vi "Periodic Tasks.vi"(8 "error in":errorcluster) -> ()   [LabVIEW 2019]
doc: "This VI runs in parallel to other tasks. It can contain as many user-defined periodic loops as you need. These can carry out PID or other sorts of timed response."
uses:
  <vilib>/Rock Robotics/WPI/Utilities/WPI_GetSetVariantRefNum.vi
  Robot Global Data.vi
  <vilib>/addons/control/pid/pid.llb/PID (DBL).vi
  <vilib>/Rock Robotics/Network Tables/NT Write Numeric Array.vi
  <vilib>/Rock Robotics/Network Tables/NT Write Number.vi
  <vilib>/Rock Robotics/Network Tables/NT Write Boolean.vi
  Secret_Control_Library_Protected/Secret_Control_Library_Protected.lvlib
  <vilib>/addons/control/pid/NI_PID_pid.lvlib
  <vilib>/Rock Robotics/WPI/ThirdParty/JAS_Junk/TrajLib/Trajectory_Library.lvlib
panel:
  in  "Speed PID":T1={"proportional gain (Kc)"=0.6, "integral time (Ti, min)"=0.015, "derivative time (Td, min)"=0.0} {"derivative time (Td, min)" format="%.3f"; "integral time (Ti, min)" format="%.3f"; "proportional gain (Kc)" format="%.3f"}
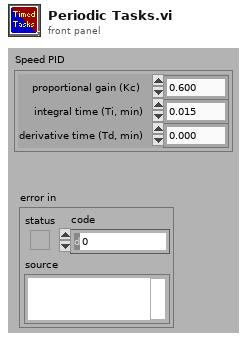
[diagram p1: front panel]
types:
  T1 = cluster{"proportional gain (Kc)":dbl, "integral time (Ti, min)":dbl, "derivative time (Td, min)":dbl}
  T2 = typedef "WPI_EncoderDevRef.ctl" = cluster{"DevStatus":errorcluster, "EncoderIndex":T3, "CounterIndex":T4, "DistancePerCount":dbl, "Decoding Type":T5}
  T3 = typedef "FPGA_EncoderIdx.ctl" = enum8{"Enc 0", "Enc 1", "Enc 2", "Enc 3", "Enc 4", "Enc 5", "Enc 6", "Enc 7", "Invalid"}
  T4 = typedef "FPGA_CounterCtrSystemIndex.ctl" = enum8{"Ctr 0", "Ctr 1", "Ctr 2", "Ctr 3", "Ctr 4", "Ctr 5", "Ctr 6", "Ctr 7", "Invalid"}
  T5 = typedef "WPI_EncoderType.ctl" = enum16{"1x", "2x", "4x"}
  T6 = typedef "WPI_GyroDevRef.ctl" = cluster{"DevStatus":errorcluster, "Analog Channel":T7, "Gain (VoltsPerDegree/Second)":dbl, "Gyro Type":enum16{"Analog", "XRS450"}, "Handle":i32, "SPI Bus":T8, "Device Found":bool, "Sample Rate":dbl, "Calibrate On Open":bool, "Offset":dbl}
  T7 = typedef "FPGA_AIChannel.ctl" = enum8{"AI 0", "AI 1", "AI 2", "AI 3", "AI MXP 0", "AI MXP 1", "AI MXP 2", "AI MXP 3", "Invalid"}
  T8 = typedef "spi_bus.ctl" = enum16{"SPI On-Board, CS0", "SPI On-Board, CS1", "SPI On-Board, CS2", "SPI On-Board, CS3", "SPI MXP", "Invalid"}
  T9 = typedef "WPI_RobotDriveDevRef.ctl" = cluster{"DevStatus":errorcluster, "Motors[]":T10[], "Square Inputs":bool, "Max Output":dbl}
  T10 = typedef "WPI_MotorControlDeviceRef.ctl" = cluster{"DeviceStatus":errorcluster, "Type":T11, "PWM":cluster{"PWM Channel":T12, "DeadBand":T13}, "CAN":cluster{"Device Number":u8, "SetOutput VI Ref":variant, "GetOutput VI Ref":variant, "Enable VI Ref":variant, "Disable VI Ref":variant, "Data":variant}, "Invert":bool, "DIO PWM":cluster{"PWM \"Enable\" Channel":T12, "DIOChannel":T14, "PWM Rate":dbl}}
  T11 = typedef "WPI_MotorControlType.ctl" = enum16{"PWM", "CAN", "DIO PWM"}
  T12 = typedef "FPGA_DIOPWMChannel.ctl" = enum8{"PWM 0", "PWM 1", "PWM 2", "PWM 3", "PWM 4", "PWM 5", "PWM 6", "PWM 7", "PWM 8", "PWM 9", "PWM MXP 0", "PWM MXP 1", "PWM MXP 2", "PWM MXP 3", "PWM MXP 4", "PWM MXP 5", "PWM MXP 6", "PWM MXP 7", "PWM MXP 8", "PWM MXP 9", "Invalid"}
  T13 = typedef "WPI_PWMDeadband.ctl" = cluster{"Name":string, "maxPositivePwm":i32, "minPositivePwm":i32, "centerPwm":i32, "maxNegativePwm":i32, "minNegativePwm":i32, "angularRange":u16}
  T14 = typedef "FPGA_DIOChannel.ctl" = enum8{"DIO 0", "DIO 1", "DIO 2", "DIO 3", "DIO 4", "DIO 5", "DIO 6", "DIO 7", "DIO 8", "DIO 9", "DIO MXP 0", "DIO MXP 1", "DIO MXP 2", "DIO MXP 3", "DIO MXP 4", "DIO MXP 5", "DIO MXP 6", "DIO MXP 7", "DIO MXP 8", "DIO MXP 9", "DIO MXP 10", "DIO MXP 11", "DIO MXP 12", "DIO MXP 13", "DIO MXP 14", "DIO MXP 15", "SPI Port CS1", "SPI Port CS2", "SPI Port CS3", "SPI Port MISO", "SPI Port MOSI", "Invalid"}
  T15 = typedef "Trajectory_Library.lvlib/SIMPLE_MOTOR_FF.ctl" = cluster{"Ks":dbl, "Kv":dbl, "Ka":dbl}
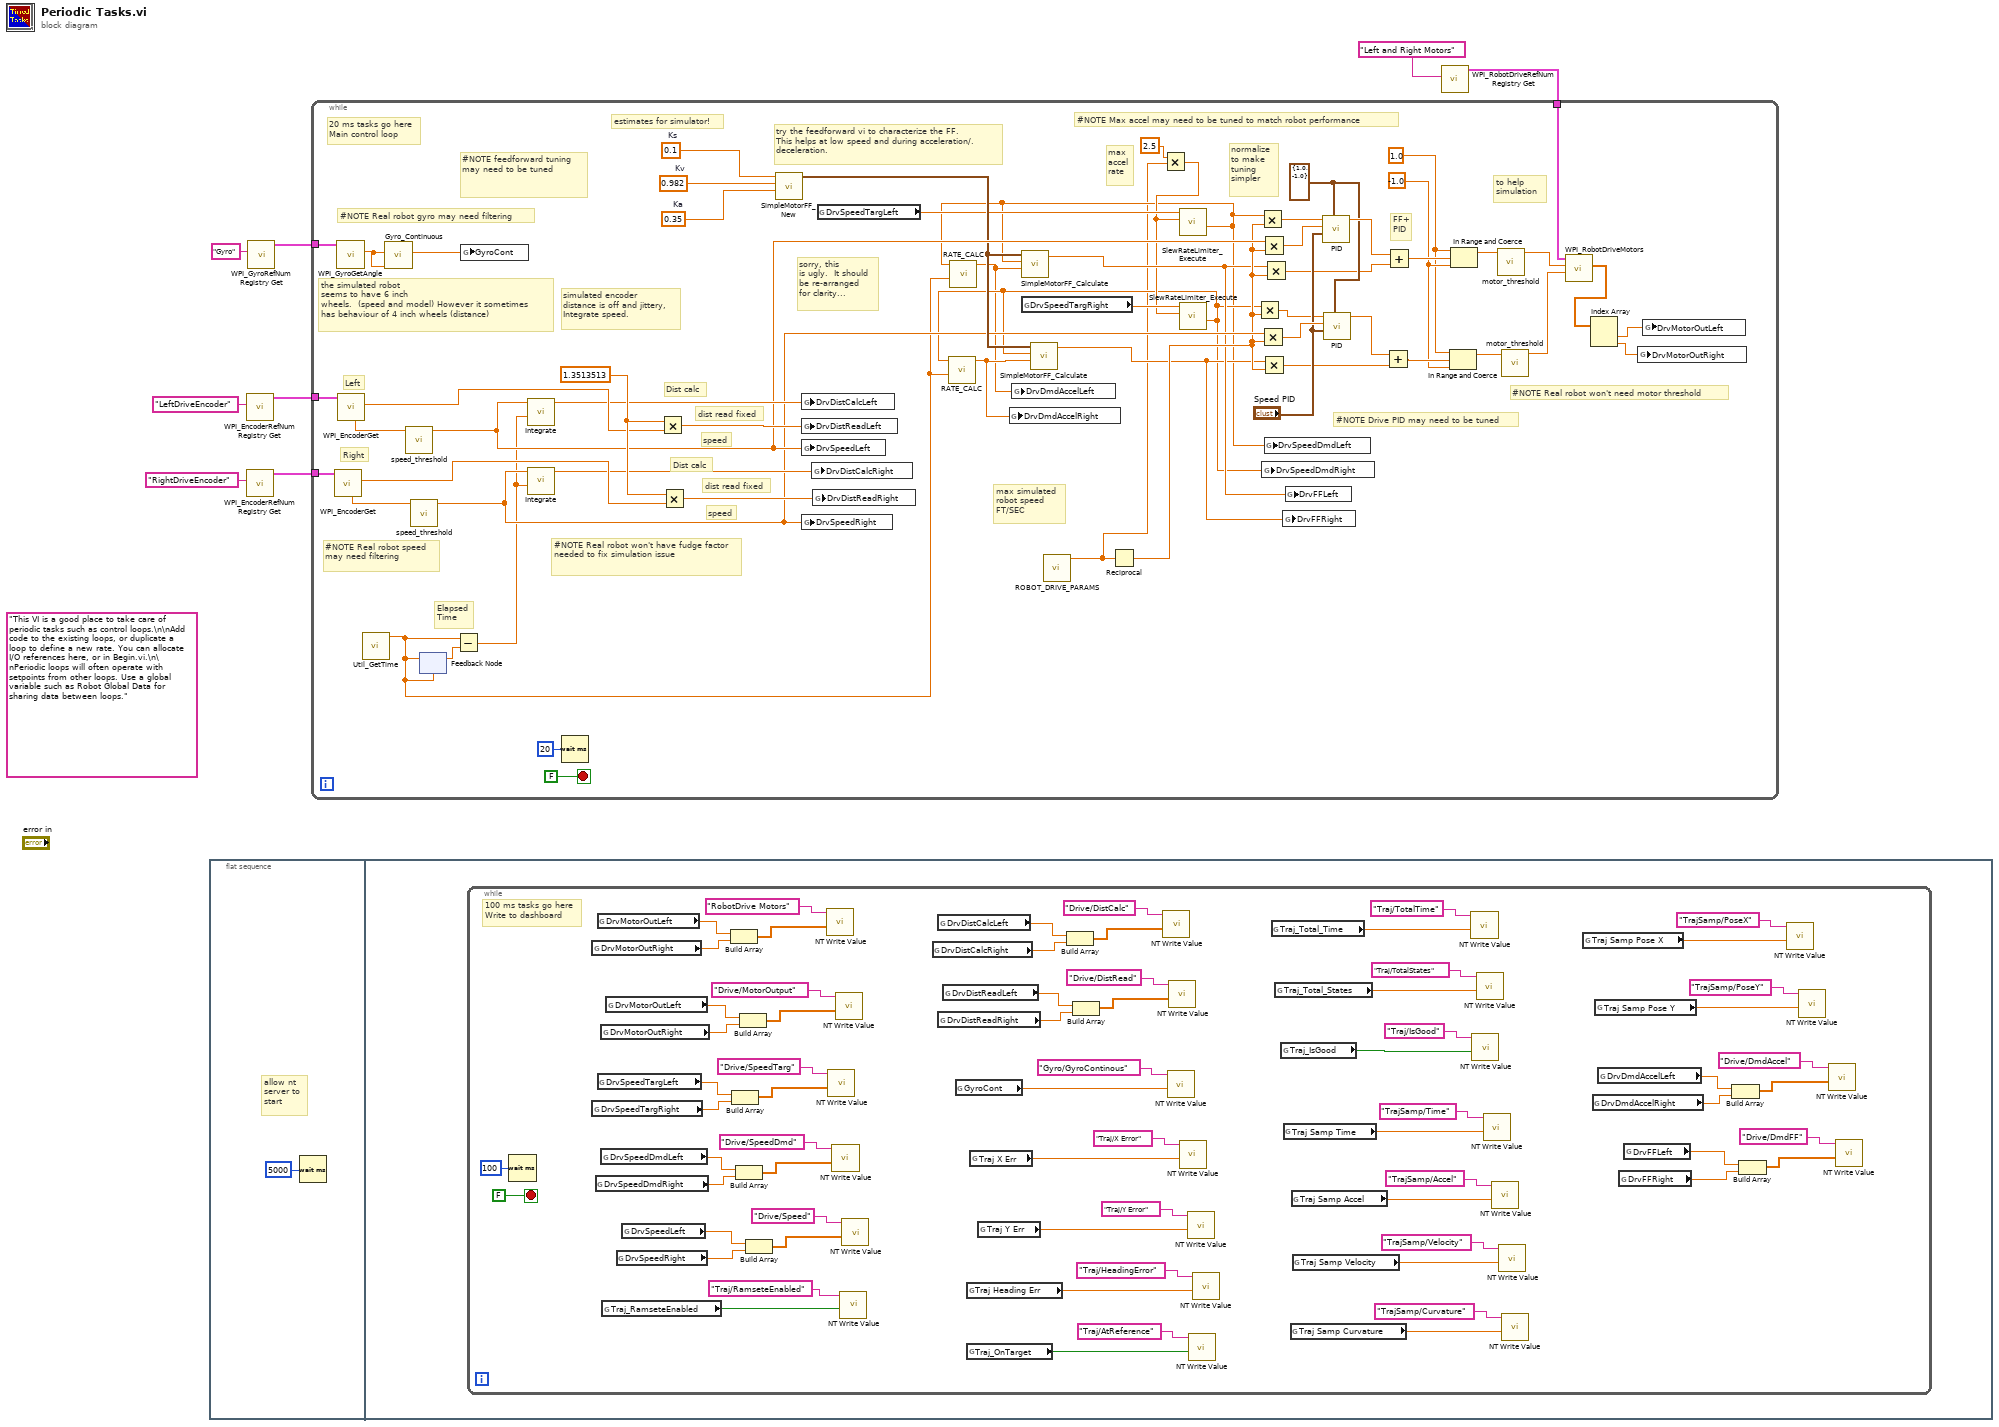
[diagram p0: block diagram]
diagram:
  (unwired) "This VI is a good place to take care of periodic tasks such as control loops.\n\nAdd code to the existing loops, or duplicate a loop to define a new rate. You can allocate I/O references here, or in Begin.vi.\n\nPeriodic loops will often operate with setpoints from other loops. Use a global variable such as Robot Global Data for sharing data between loops."
  n1 = flat-sequence {
    frame #0 {
      # "allow nt\nserver to \nstart"
      n2 = Wait (ms)(milliseconds to wait=u32 5000) -> ()  [unwired: 1 out]
    }
    frame #1 {
      n3 = while {
        stop <- FALSE stop-if-true
        # "100 ms tasks go here\nWrite to dashboard"
        n4 = Wait (ms)(milliseconds to wait=u32 100) -> ()  [unwired: 1 out]
        n5 = global read "Robot Global Data.vi" "DrvMotorOutRight"() -> (w74:dbl)
        n6 = global read "Robot Global Data.vi" "DrvSpeedTargRight"() -> (w66:dbl)
        n7 = global read "Robot Global Data.vi" "DrvSpeedDmdRight"() -> (w62:dbl)
        n8 = global read "Robot Global Data.vi" "DrvMotorOutLeft"() -> (w75:dbl)
        n9 = global read "Robot Global Data.vi" "DrvSpeedTargLeft"() -> (w67:dbl)
        n10 = global read "Robot Global Data.vi" "DrvMotorOutRight"() -> (w70:dbl)
        n11 = global read "Robot Global Data.vi" "DrvSpeedDmdLeft"() -> (w63:dbl)
        n12 = global read "Robot Global Data.vi" "Traj_RamseteEnabled"() -> (w11:bool)
        n13 = global read "Robot Global Data.vi" "DrvMotorOutLeft"() -> (w71:dbl)
        n14 = global read "Robot Global Data.vi" "DrvSpeedRight"() -> (w58:dbl)
        n15 = global read "Robot Global Data.vi" "DrvSpeedLeft"() -> (w59:dbl)
        n16 = Build Array(w75, w74) -> (w73:dbl[])
        n17 = Build Array(w67, w66) -> (w65:dbl[])
        n18 = Build Array(w63, w62) -> (w61:dbl[])
        n19 = Build Array(w71, w70) -> (w69:dbl[])
        n20 = Build Array(w59, w58) -> (w57:dbl[])
        n21 = call-poly <vilib>:"NT Write Value.vi"("Numeric Array"=w73, "Name"="RobotDrive Motors") -> ()  [unwired: 9 in, 1 out]
        n22 = call-poly <vilib>:"NT Write Value.vi"("Numeric Array"=w65, "Name"="Drive/SpeedTarg") -> ()  [unwired: 9 in, 1 out]
        n23 = call-poly <vilib>:"NT Write Value.vi"("Numeric Array"=w61, "Name"="Drive/SpeedDmd") -> ()  [unwired: 9 in, 1 out]
        n24 = call-poly <vilib>:"NT Write Value.vi"("Numeric Array"=w69, "Name"="Drive/MotorOutput") -> ()  [unwired: 9 in, 1 out]
        n25 = call-poly <vilib>:"NT Write Value.vi"("Boolean"=w11, "Name"="Traj/RamseteEnabled") -> ()  [unwired: 9 in, 1 out]
        n26 = call-poly <vilib>:"NT Write Value.vi"("Numeric Array"=w57, "Name"="Drive/Speed") -> ()  [unwired: 9 in, 1 out]
        n27 = global read "Robot Global Data.vi" "DrvDistCalcRight"() -> (w54:dbl)
        n28 = global read "Robot Global Data.vi" "DrvDistCalcLeft"() -> (w55:dbl)
        n29 = global read "Robot Global Data.vi" "DrvDistReadRight"() -> (w50:dbl)
        n30 = global read "Robot Global Data.vi" "DrvDistReadLeft"() -> (w51:dbl)
        n31 = global read "Robot Global Data.vi" "GyroCont"() -> (w46:dbl)
        n32 = global read "Robot Global Data.vi" "Traj Heading Err"() -> (w40:dbl)
        n33 = global read "Robot Global Data.vi" "Traj_OnTarget"() -> (w38:bool)
        n34 = global read "Robot Global Data.vi" "Traj X Err"() -> (w44:dbl)
        n35 = global read "Robot Global Data.vi" "Traj Y Err"() -> (w42:dbl)
        n36 = Build Array(w55, w54) -> (w53:dbl[])
        n37 = Build Array(w51, w50) -> (w49:dbl[])
        n38 = call-poly <vilib>:"NT Write Value.vi"("Numeric Array"=w53, "Name"="Drive/DistCalc") -> ()  [unwired: 9 in, 1 out]
        n39 = call-poly <vilib>:"NT Write Value.vi"("Numeric"=w46, "Name"="Gyro/GyroContinous") -> ()  [unwired: 9 in, 1 out]
        n40 = call-poly <vilib>:"NT Write Value.vi"("Numeric Array"=w49, "Name"="Drive/DistRead") -> ()  [unwired: 9 in, 1 out]
        n41 = call-poly <vilib>:"NT Write Value.vi"("Numeric"=w44, "Name"="Traj/X Error") -> ()  [unwired: 9 in, 1 out]
        n42 = call-poly <vilib>:"NT Write Value.vi"("Numeric"=w42, "Name"="Traj/Y Error") -> ()  [unwired: 9 in, 1 out]
        n43 = call-poly <vilib>:"NT Write Value.vi"("Boolean"=w38, "Name"="Traj/AtReference") -> ()  [unwired: 9 in, 1 out]
        n44 = call-poly <vilib>:"NT Write Value.vi"("Numeric"=w40, "Name"="Traj/HeadingError") -> ()  [unwired: 9 in, 1 out]
        n45 = global read "Robot Global Data.vi" "Traj_Total_Time"() -> (w36:dbl)
        n46 = global read "Robot Global Data.vi" "Traj_Total_States"() -> (w34:dbl)
        n47 = global read "Robot Global Data.vi" "Traj_IsGood"() -> (w32:bool)
        n48 = global read "Robot Global Data.vi" "Traj Samp Time"() -> (w30:dbl)
        n49 = global read "Robot Global Data.vi" "Traj Samp Curvature"() -> (w24:dbl)
        n50 = global read "Robot Global Data.vi" "Traj Samp Accel"() -> (w28:dbl)
        n51 = global read "Robot Global Data.vi" "Traj Samp Velocity"() -> (w26:dbl)
        n52 = call-poly <vilib>:"NT Write Value.vi"("Numeric"=w36, "Name"="Traj/TotalTime") -> ()  [unwired: 9 in, 1 out]
        n53 = call-poly <vilib>:"NT Write Value.vi"("Boolean"=w32, "Name"="Traj/IsGood") -> ()  [unwired: 9 in, 1 out]
        n54 = call-poly <vilib>:"NT Write Value.vi"("Numeric"=w34, "Name"="Traj/TotalStates") -> ()  [unwired: 9 in, 1 out]
        n55 = call-poly <vilib>:"NT Write Value.vi"("Numeric"=w30, "Name"="TrajSamp/Time") -> ()  [unwired: 9 in, 1 out]
        n56 = call-poly <vilib>:"NT Write Value.vi"("Numeric"=w28, "Name"="TrajSamp/Accel") -> ()  [unwired: 9 in, 1 out]
        n57 = call-poly <vilib>:"NT Write Value.vi"("Numeric"=w26, "Name"="TrajSamp/Velocity") -> ()  [unwired: 9 in, 1 out]
        n58 = call-poly <vilib>:"NT Write Value.vi"("Numeric"=w24, "Name"="TrajSamp/Curvature") -> ()  [unwired: 9 in, 1 out]
        n59 = global read "Robot Global Data.vi" "Traj Samp Pose X"() -> (w22:dbl)
        n60 = global read "Robot Global Data.vi" "DrvDmdAccelRight"() -> (w18:dbl)
        n61 = global read "Robot Global Data.vi" "Traj Samp Pose Y"() -> (w20:dbl)
        n62 = global read "Robot Global Data.vi" "DrvDmdAccelLeft"() -> (w19:dbl)
        n63 = global read "Robot Global Data.vi" "DrvFFRight"() -> (w14:dbl)
        n64 = global read "Robot Global Data.vi" "DrvFFLeft"() -> (w15:dbl)
        n65 = Build Array(w19, w18) -> (w17:dbl[])
        n66 = Build Array(w15, w14) -> (w13:dbl[])
        n67 = call-poly <vilib>:"NT Write Value.vi"("Numeric"=w22, "Name"="TrajSamp/PoseX") -> ()  [unwired: 9 in, 1 out]
        n68 = call-poly <vilib>:"NT Write Value.vi"("Numeric"=w20, "Name"="TrajSamp/PoseY") -> ()  [unwired: 9 in, 1 out]
        n69 = call-poly <vilib>:"NT Write Value.vi"("Numeric Array"=w17, "Name"="Drive/DmdAccel") -> ()  [unwired: 9 in, 1 out]
        n70 = call-poly <vilib>:"NT Write Value.vi"("Numeric Array"=w13, "Name"="Drive/DmdFF") -> ()  [unwired: 9 in, 1 out]
      }
    }
  }
  n71 = call <vilib>:"WPI_EncoderRefNum Registry Get.vi"("refnum name"="LeftDriveEncoder") -> ("EncoderDevRef"=w6:T2)  [unwired: 9 in, 1 out]
  n72 = call <vilib>:"WPI_EncoderRefNum Registry Get.vi"("refnum name"="RightDriveEncoder") -> ("EncoderDevRef"=w7:T2)  [unwired: 9 in, 1 out]
  n73 = call <vilib>:"WPI_GyroRefNum Registry Get.vi"("refnum name"="Gyro") -> ("GyroDevRef"=w2:T6)  [unwired: 9 in, 1 out]
  n74 = call <vilib>:"WPI_RobotDriveRefNum Registry Get.vi"("refnum name"="Left and Right Motors") -> ("RobotDriveDevRef"=w1:T9)  [unwired: 1 in, 9 out]
  n75 = while {
    tunnel: w7 -> [w131]
    tunnel: w6 -> [w130]
    tunnel: w2 -> [w128]
    tunnel: w1 -> [w114]
    stop <- FALSE stop-if-true
    w97 = 0.35  # Ka
    w98 = 0.982  # Kv
    w99 = 0.1  # Ks
    w123 = -1.0 ("lower limit")
    w122 = 1.0 ("upper limit")
    w120 = cluster{"output high":dbl, "output low":dbl} {"output high"=1.0, "output low"=-1.0} ("output range")
    w134 = 1.3513513
    # "#NOTE Real robot won't need motor threshold"
    # "#NOTE Real robot won't have fudge factor needed to fix simulation issue"
    # "#NOTE Max accel may need to be tuned to match robot performance"
    # "#NOTE Drive PID may need to be tuned"
    # "#NOTE feedforward tuning may need to be tuned"
    # "Elapsed\nTime"
    # "estimates for simulator!"
    # "sorry, this\nis ugly.  It should\nbe re-arranged\nfor clarity..."
    # "try the feedforward vi to characterize the FF.\nThis helps at low speed and during acceleration/.\ndeceleration."
    # "to help\nsimulation"
    # "#NOTE Real robot speed may need filtering"
    # "max simulated\nrobot speed\nFT/SEC"
    # "max\naccel\nrate"
    # "normalize\nto make\ntuning\nsimpler"
    # "FF+\nPID"
    # "#NOTE Real robot gyro may need filtering"
    # "Right"
    # "Left"
    # "the simulated robot\nseems to have 6 inch\nwheels.  (speed and model) However it sometimes\nhas behaviour of 4 inch wheels (distance)"
    # "speed"
    # "dist read fixed"
    # "Dist calc"
    # "speed"
    # "dist read fixed"
    # "Dist calc"
    # "simulated encoder\ndistance is off and jittery,\nIntegrate speed."
    # "20 ms tasks go here\nMain control loop"
    n76 = call <vilib>:"WPI_EncoderGet.vi"("EncoderDevRef"=w131) -> ("Distance"=w132:dbl, "Rate"=w105:dbl)  [unwired: 5 in, 4 out]
    n77 = call <vilib>:"WPI_GyroGetAngle.vi"("GyroDevRef"=w128) -> ("Angle"=w129:dbl)  [unwired: 7 in, 3 out]
    n78 = call <vilib>:"WPI_EncoderGet.vi"("EncoderDevRef"=w130) -> ("Distance"=w133:dbl, "Rate"=w106:dbl)  [unwired: 5 in, 4 out]
    n79 = call <vilib>:"Util_GetTime.vi"() -> ("FPGA_Time_Seconds"=w79:dbl)  [unwired: 10 in, 1 out]
    n80 = call "Gyro_Continuous.vi"("GyroInitial"=w129, "GyroInput"=w129) -> ("GyroContinuous"=w100:dbl)  [unwired: 9 in]
    n81 = call "speed_threshold.vi"("SPEED IN"=w106) -> ("SPEED OUT"=w96:dbl)  [unwired: 10 in]
    n82 = call "speed_threshold.vi"("SPEED IN"=w105) -> ("SPEED OUT"=w94:dbl)  [unwired: 10 in]
    n83 = feedback-in #1(w79) -> ()
    n84 = feedback #1(w79) -> (w85:dbl)
    n85 = Subtract(x=w79, y=w85) -> (x-y=w84:dbl)
    n86 = global write "Robot Global Data.vi" "GyroCont"(w100) -> ()
    n87 = call "Integrate.vi"("Elapsed Sec"=w84, "Rate"=w96) -> ("DIST"=w113:dbl)  [unwired: 9 in]
    n88 = call "Integrate.vi"("Elapsed Sec"=w84, "Rate"=w94) -> ("DIST"=w111:dbl)  [unwired: 9 in]
    n89 = Wait (ms)(milliseconds to wait=u32 20) -> ()  [unwired: 1 out]
    n90 = Multiply(x=w134, y=w133) -> (x*y=w112:dbl)
    n91 = Multiply(x=w134, y=w132) -> (x*y=w110:dbl)
    n92 = call <vilib>:"SimpleMotorFF_New.vi"("Ka"=w97, "Kv"=w98, "Ks"=w99) -> ("SIMPLE_MOTOR_FF"=w95:T15)  [unwired: 8 in]
    n93 = global write "Robot Global Data.vi" "DrvDistCalcLeft"(w113) -> ()
    n94 = global write "Robot Global Data.vi" "DrvDistReadLeft"(w112) -> ()
    n95 = global write "Robot Global Data.vi" "DrvSpeedLeft"(w96) -> ()
    n96 = global write "Robot Global Data.vi" "DrvSpeedRight"(w94) -> ()
    n97 = global write "Robot Global Data.vi" "DrvDistCalcRight"(w111) -> ()
    n98 = global write "Robot Global Data.vi" "DrvDistReadRight"(w110) -> ()
    n99 = global read "Robot Global Data.vi" "DrvSpeedTargLeft"() -> (w88:dbl)
    n100 = global read "Robot Global Data.vi" "DrvSpeedTargRight"() -> (w87:dbl)
    n101 = call "ROBOT_DRIVE_PARAMS.vi"() -> ("Max Speed Ft/Sec"=w78:dbl)  [unwired: 10 in, 1 out]
    n102 = Reciprocal(x=w78) -> (1/x=w93:dbl)
    n103 = Multiply(x=2.5, y=w78) -> (x*y=w86:dbl)
    n104 = call <vilib>:"SlewRateLimiter_Execute.vi"("Rate"=w86, "Input"=w88) -> ("Output"=w80:dbl)  [unwired: 8 in, 1 out]
    n105 = call "RATE_CALC.vi"("Time"=w79, "Input"=w80) -> ("Output"=w81:dbl)  [unwired: 9 in]
    n106 = global write "Robot Global Data.vi" "DrvDmdAccelLeft"(w81) -> ()
    n107 = call <vilib>:"SimpleMotorFF_Calculate.vi"("Accel"=w81, "Vel"=w80, "SIMPLE_MOTOR_FF"=w95) -> ("FeedForward"=w90:dbl)  [unwired: 8 in]
    n108 = call <vilib>:"SlewRateLimiter_Execute.vi"("Rate"=w86, "Input"=w87) -> ("Output"=w82:dbl)  [unwired: 8 in, 1 out]
    n109 = call "RATE_CALC.vi"("Time"=w79, "Input"=w82) -> ("Output"=w83:dbl)  [unwired: 9 in]
    n110 = global write "Robot Global Data.vi" "DrvDmdAccelRight"(w83) -> ()
    n111 = call <vilib>:"SimpleMotorFF_Calculate.vi"("Accel"=w83, "Vel"=w82, "SIMPLE_MOTOR_FF"=w95) -> ("FeedForward"=w89:dbl)  [unwired: 8 in]
    n112 = Multiply(x=w82, y=w93) -> (x*y=w117:dbl)
    n113 = Multiply(x=w80, y=w93) -> (x*y=w116:dbl)
    n114 = Multiply(x=w94, y=w93) -> (x*y=w121:dbl)
    n115 = Multiply(x=w96, y=w93) -> (x*y=w118:dbl)
    n116 = Multiply(x=w89, y=w93) -> (x*y=w91:dbl)
    n117 = global write "Robot Global Data.vi" "DrvSpeedDmdRight"(w82) -> ()
    n118 = Multiply(x=w90, y=w93) -> (x*y=w92:dbl)
    n119 = global write "Robot Global Data.vi" "DrvSpeedDmdLeft"(w80) -> ()
    n120 = global write "Robot Global Data.vi" "DrvFFRight"(w89) -> ()
    n121 = global write "Robot Global Data.vi" "DrvFFLeft"(w90) -> ()
    n122 = call-poly <vilib>:"PID.vi"("output range"=w120, "PID gains"="Speed PID", "process variable"=w118, "setpoint"=w116) -> ("output"=w127:dbl)  [unwired: 6 in, 1 out]
    n123 = call-poly <vilib>:"PID.vi"("output range"=w120, "PID gains"="Speed PID", "process variable"=w121, "setpoint"=w117) -> ("output"=w125:dbl)  [unwired: 6 in, 1 out]
    n124 = Add(x=w125, y=w91) -> (x+y=w124:dbl)
    n125 = Add(x=w127, y=w92) -> (x+y=w126:dbl)
    n126 = In Range and Coerce(upper limit=w122, x=w124, lower limit=w123) -> (coerced(x)=w102:dbl)  [unwired: 1 out]
    n127 = In Range and Coerce(upper limit=w122, x=w126, lower limit=w123) -> (coerced(x)=w103:dbl)  [unwired: 1 out]
    n128 = call "motor_threshold.vi"("motor in"=w103) -> ("motor out"=w104:dbl)  [unwired: 10 in]
    n129 = call "motor_threshold.vi"("motor in"=w102) -> ("motor out"=w101:dbl)  [unwired: 10 in]
    n130 = call <vilib>:"WPI_RobotDriveMotors.vi"("RightSpeed"=w101, "LeftSpeed"=w104, "RobotDriveDevRef"=w114) -> ("Motor Values"=w109:dbl[])  [unwired: 6 in, 2 out]
    n131 = Index Array(array=w109) -> (element #1=w108:dbl, element #2=w107:dbl)  [unwired: 2 in]
    n132 = global write "Robot Global Data.vi" "DrvMotorOutRight"(w107) -> ()
    n133 = global write "Robot Global Data.vi" "DrvMotorOutLeft"(w108) -> ()
  }
